vi "GLdrv_IF_IP.vi"(0 "Connection ID":T1, 5 "IP":string, 11 "error in (no error)":errorcluster, 13 "Query(f)":bool) -> (4 "Connection ID Out":T1, 6 "IP out":string, 15 "error out":errorcluster)   [LabVIEW 2017, in "GL860_Driver.lvlib"]
doc: "TCP/IP、UDP/IP用IPアドレスを設定します\n本体の再起動後に設定が反映されます\n※DHCP ON時は自動取得した値を参照できます。\n<NR1>: 0-255\n例) :IF:IP 192,168,0,1\n※各数値の区切りはピリオド(.)ではなくカンマ(,)です。ご注意ください。"
uses:
  GL860_Driver.lvlib
  ConnectionID.ctl
  GLdrv_RW.ctl
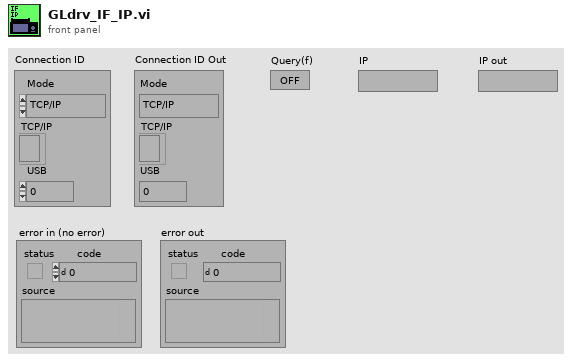
[diagram p1: front panel]
types:
  T1 = typedef "ConnectionID.ctl" = cluster{"Mode":enum16{"TCP/IP", "USB"}, "TCP/IP":refnum<k5>, "USB":i32}
  T2 = typedef "GLdrv_RW.ctl" = enum16{"Auto", "Read", "Write", "Buffer"}
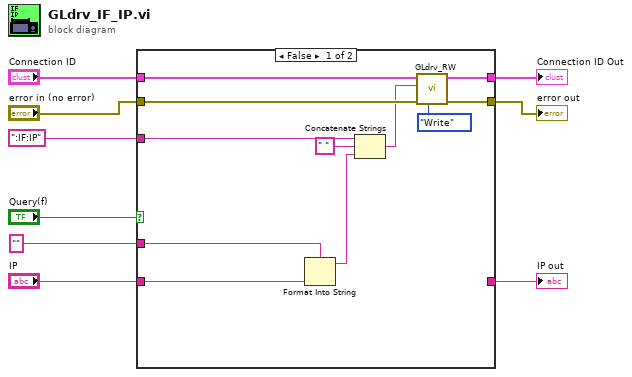
[diagram p0: block diagram]
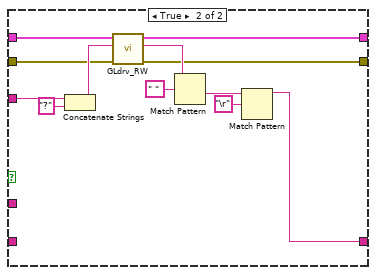
[diagram p2: hidden frame]
diagram:
  n1 = case shown="FALSE" "Query(f)" {
    tunnel: ":IF:IP" ("Command") -> [w20 w29]
    tunnel: [w15 w22] -> w9
    tunnel: [w17 w26] -> w8
    tunnel: "Connection ID" -> [w18 w27]
    tunnel: "error in (no error)" -> [w16 w23]
    tunnel: "IP" -> [w11 _]
    tunnel: [_ w21] -> w1
    tunnel: "" ("Param") -> [w10 _]
    frame False {
      n2 = Format Into String(format string=w10, w11) -> (resulting string=w12:string)  [unwired: 2 in, 1 out]
      n3 = Concatenate Strings(w20, " " ("string"), w12) -> (w14:string)
      n4 = call "GLdrv_RW.vi"("Mode(read)"=GLdrv_RW."Write", "error in (no error)"=w16, "data in"=w14, "Connection ID"=w18) -> ("error out"=w15:errorcluster, "Connection ID Out"=w17:T1)  [unwired: 3 in, 3 out]
    }
    frame True {
      n5 = Concatenate Strings(w29, "?" ("string")) -> (w25:string)
      n6 = call "GLdrv_RW.vi"("error in (no error)"=w23, "data in"=w25, "Connection ID"=w27) -> ("error out"=w22:errorcluster, "data out"=w24:string, "Connection ID Out"=w26:T1)  [unwired: 4 in, 2 out]
      n7 = Match Pattern(string=w24, regular expression=" " ("search string/char (-)")) -> (after substring=w30:string)  [unwired: 4 out]
      n8 = Match Pattern(string=w30, regular expression="\r") -> (before substring=w21:string)  [unwired: 4 out]
    }
  }
  "Connection ID Out" <- w8
  "error out" <- w9
  "IP out" <- w1
